vi "Auto1RecycleBin.vi"(8 "error in":errorcluster) -> ()   [LabVIEW 2014]
uses:
  <vilib>/Rock Robotics/WPI/DriverStation/WPI_DriverStationRobotMode2.ctl
  LowerLiftAndOpenArms.ctl
  Robot Global Data.vi
  Gantry/GantryGlobals.vi
  AutomationGlobals.vi
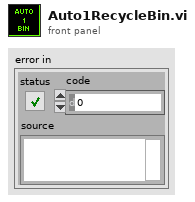
[diagram p1: front panel]
types:
  T1 = enum16{"WaitForInput", "GantryOut", "Lift", "Forward", "Autostack", "Left", "PutToteDown", "GrabBarrelLift", "Right", "Forward2", "Done"}
  T2 = typedef "WPI_DriverStationRobotMode2.ctl" = enum16{"Autonomous Disabled", "Autonomous Enabled", "Teleop Disabled", "Teleop Enabled", "Disconnected", "Finish", "Test Disabled", "Test Enabled", "Emergency Stopped"}
  T3 = typedef "LowerLiftAndOpenArms.ctl" = enum16{"WaitingForInput", "LowerLift", "OpenArms", "LowerLiftMore", "CloseArms", "RaiseLift", "StopArms"}
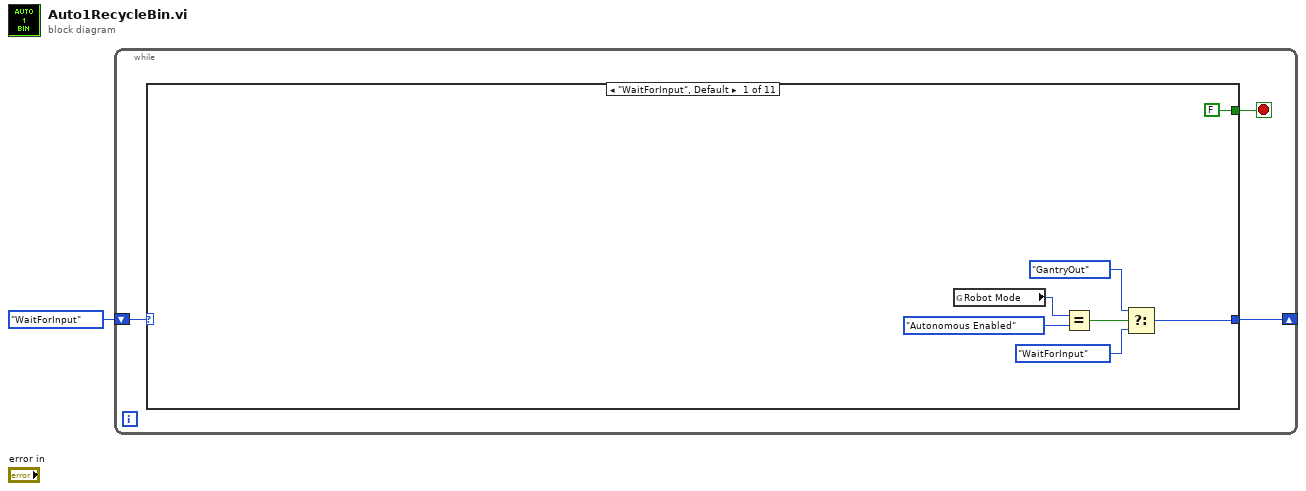
[diagram p0: block diagram]
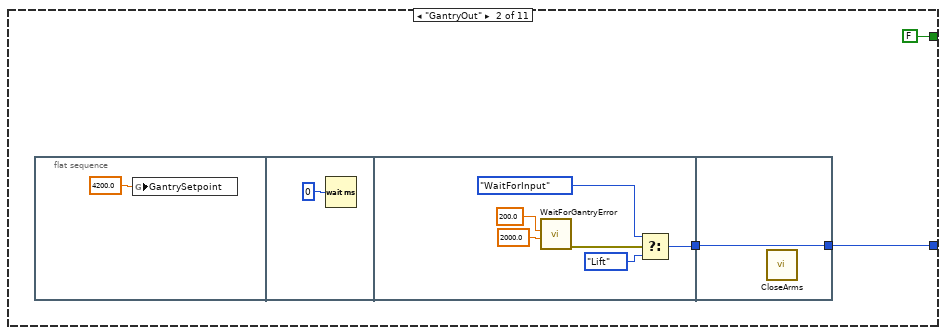
[diagram p2: hidden frame]
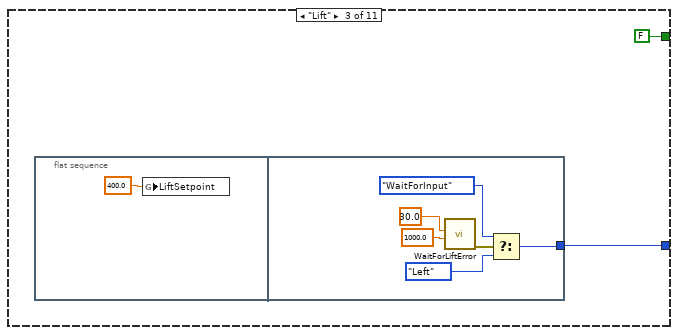
[diagram p3: hidden frame]
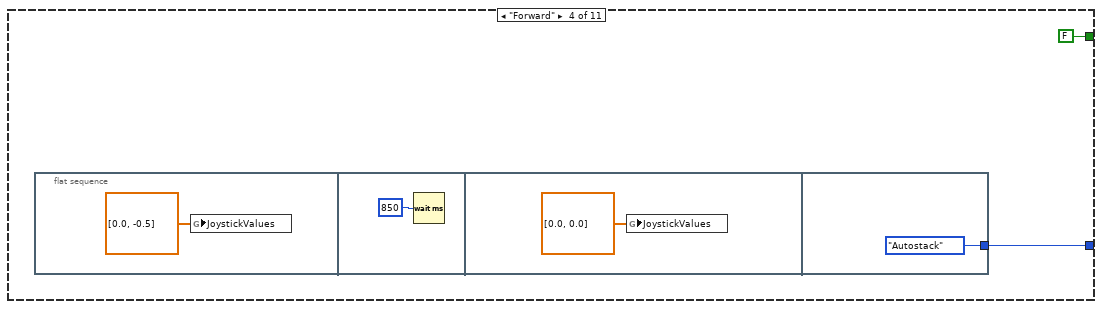
[diagram p4: hidden frame]
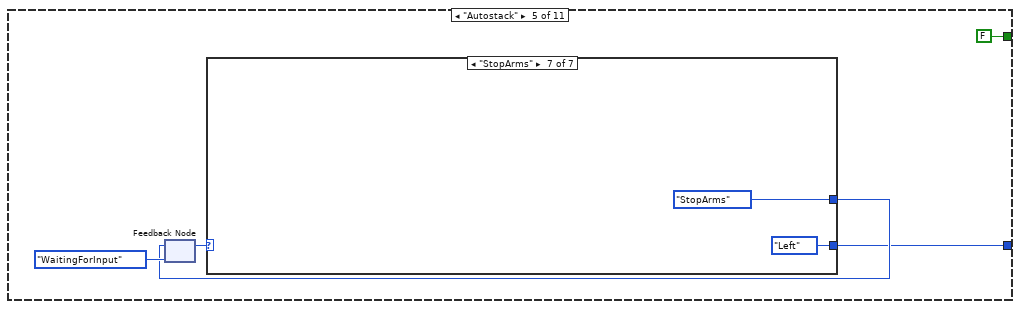
[diagram p5: hidden frame]
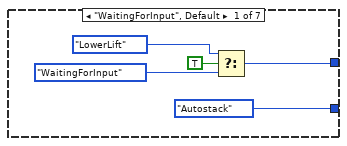
[diagram p6: hidden frame]
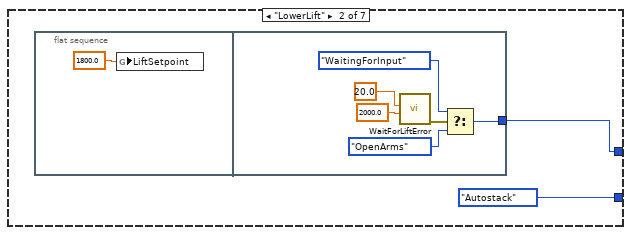
[diagram p7: hidden frame]
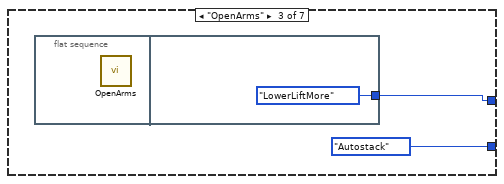
[diagram p8: hidden frame]
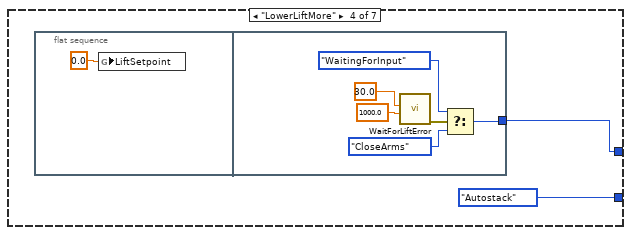
[diagram p9: hidden frame]
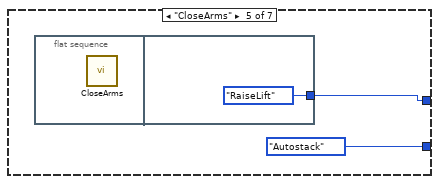
[diagram p10: hidden frame]
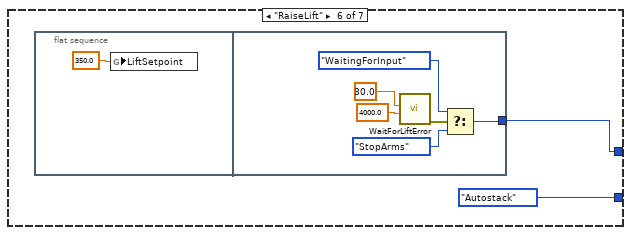
[diagram p11: hidden frame]
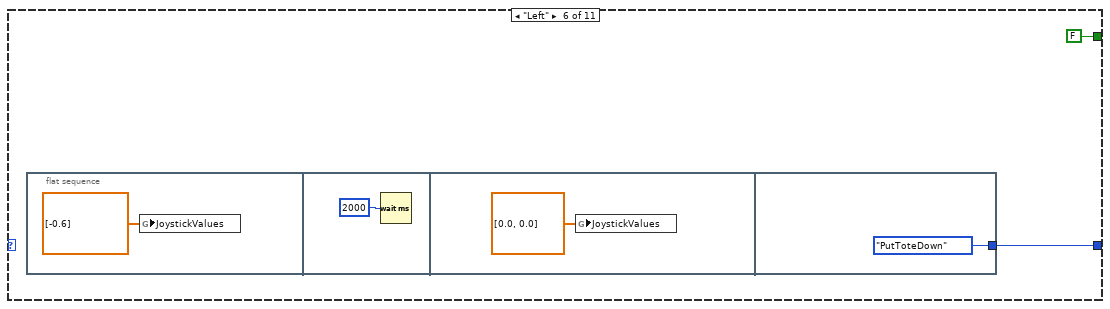
[diagram p12: hidden frame]
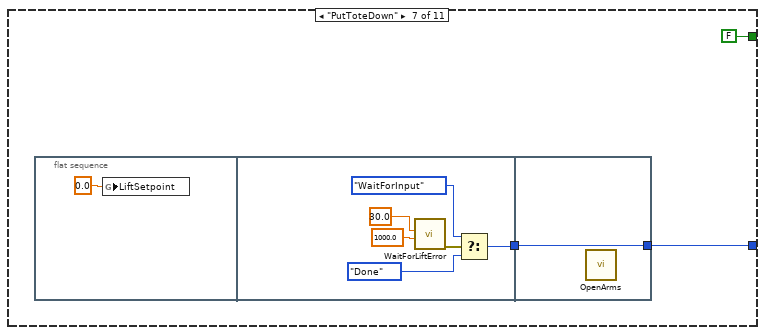
[diagram p13: hidden frame]
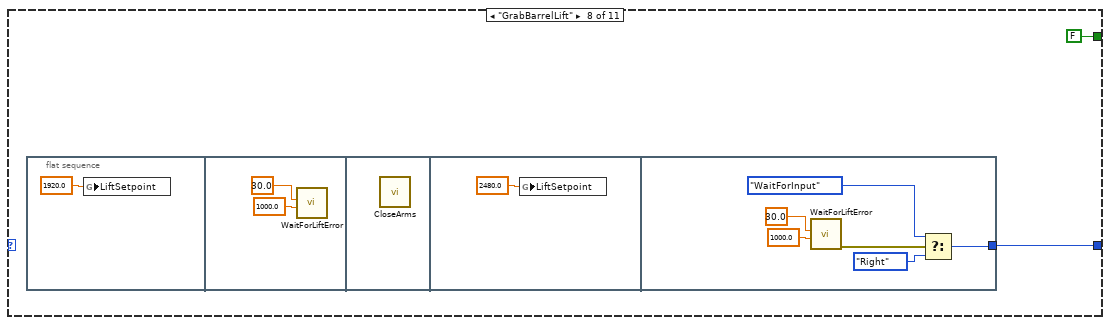
[diagram p14: hidden frame]
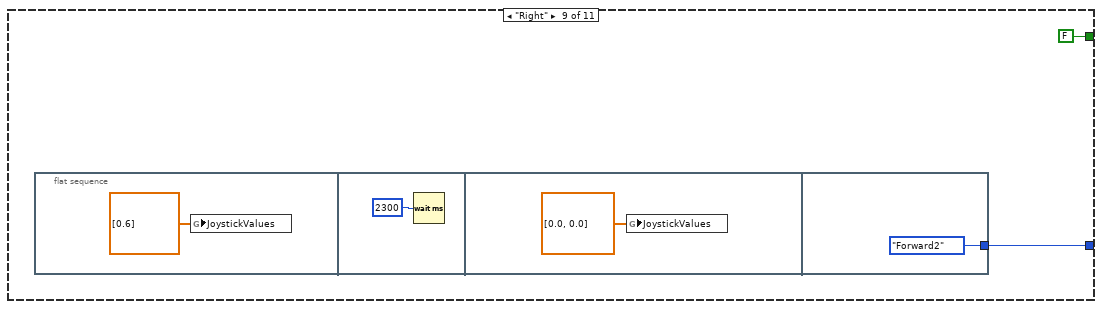
[diagram p15: hidden frame]
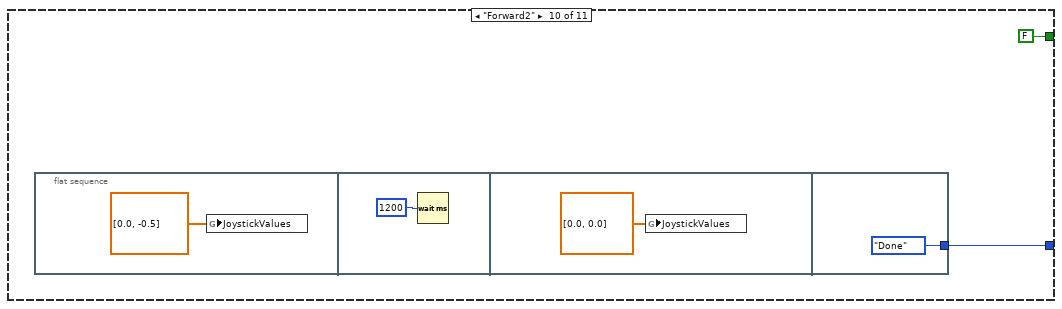
[diagram p16: hidden frame]
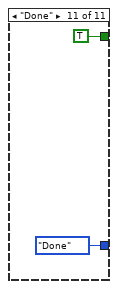
[diagram p17: hidden frame]
diagram:
  n1 = while {
    shift-right: [w3] -> _
    shift-left: T1."WaitForInput" ("Enum") -> [w4]
    stop <- w2 stop-if-true
    n2 = case shown="\"WaitForInput\", Default" w4 {
      tunnel: [w8 w14 w25 w33 w39 w84 w91 w101 w113 w120 T1."Done" ("Enum")] -> w3
      tunnel: [FALSE FALSE FALSE FALSE FALSE FALSE FALSE FALSE FALSE FALSE TRUE] -> w2
      frame "WaitForInput", Default {
        n3 = global read "Robot Global Data.vi" "Robot Mode"() -> (w11:T2)
        n4 = Equal?(x=w11, y=WPI_DriverStationRobotMode2."Autonomous Enabled") -> (x = y?=w9:bool)
        n5 = Select(t=T1."GantryOut" ("Enum"), s=w9, f=T1."WaitForInput" ("Enum")) -> (s? t:f=w8:T1)
      }
      frame "GantryOut" {
        n6 = flat-sequence {
          tunnel: [w19] -> w12
          tunnel: [w23] -> w14
          tunnel: w12 -> [w23]
          frame #0 {
            n7 = global write "GantryGlobals.vi" "GantrySetpoint"(4200.0 ("GantrySetpoint")) -> ()
          }
          frame #1 {
            n8 = Wait (ms)(milliseconds to wait=u32 0) -> ()  [unwired: 1 out]
          }
          frame #2 {
            n9 = call "WaitForGantryError.vi"("Timeout (ms)"=2000.0, "AllowedError"=200.0) -> ("error out"=w20:errorcluster)  [unwired: 9 in]
            n10 = Select(t=T1."WaitForInput" ("Enum"), s=w20, f=T1."Lift" ("Enum")) -> (s? t:f=w19:T1)
          }
          frame #3 {
            n11 = call "CloseArms.vi"() -> ()  [unwired: 12 in]
          }
        }
      }
      frame "Lift" {
        n12 = flat-sequence {
          tunnel: [w29] -> w25
          frame #0 {
            n13 = global write "GantryGlobals.vi" "LiftSetpoint"(400.0 ("LiftSetpoint")) -> ()
          }
          frame #1 {
            n14 = call "WaitForLiftError.vi"("Timeout (ms)"=1000.0, "AllowedError"=30.0) -> ("error out"=w32:errorcluster)  [unwired: 9 in]
            n15 = Select(t=T1."WaitForInput" ("Enum"), s=w32, f=T1."Left" ("Enum")) -> (s? t:f=w29:T1)
          }
        }
      }
      frame "Forward" {
        n16 = flat-sequence {
          tunnel: [T1."Autostack" ("Enum")] -> w33
          frame #0 {
            n17 = global write "AutomationGlobals.vi" "JoystickValues"(dbl[] [0.0, -0.5] ("s? t:f")) -> ()
          }
          frame #1 {
            n18 = Wait (ms)(milliseconds to wait=u32 850) -> ()  [unwired: 1 out]
          }
          frame #2 {
            n19 = global write "AutomationGlobals.vi" "JoystickValues"(dbl[] [0.0, 0.0] ("s? t:f")) -> ()
          }
          frame #3 {
          }
        }
      }
      frame "Autostack" {
        n20 = feedback #1(LowerLiftAndOpenArms."WaitingForInput" ("LowerAndOpen")) -> (w41:T3)
        n21 = case shown="\"StopArms\"" w41 {
          tunnel: [w46 w50 w59 w62 w71 w74 LowerLiftAndOpenArms."StopArms" ("LowerAndOpen")] -> w40
          tunnel: [T1."Autostack" ("Enum") T1."Autostack" ("Enum") T1."Autostack" ("Enum") T1."Autostack" ("Enum") T1."Autostack" ("Enum") T1."Autostack" ("Enum") T1."Left" ("Enum")] -> w39
          frame "WaitingForInput", Default {
            n22 = Select(t=LowerLiftAndOpenArms."LowerLift" ("LowerAndOpen"), s=TRUE, f=LowerLiftAndOpenArms."WaitingForInput" ("LowerAndOpen")) -> (s? t:f=w46:T3)
          }
          frame "LowerLift" {
            n23 = flat-sequence {
              tunnel: [w52] -> w50
              frame #0 {
                n24 = global write "GantryGlobals.vi" "LiftSetpoint"(1800.0 ("LiftSetpoint")) -> ()
              }
              frame #1 {
                n25 = call "WaitForLiftError.vi"("Timeout (ms)"=2000.0, "AllowedError"=20.0) -> ("error out"=w55:errorcluster)  [unwired: 9 in]
                n26 = Select(t=LowerLiftAndOpenArms."WaitingForInput" ("LowerAndOpen"), s=w55, f=LowerLiftAndOpenArms."OpenArms" ("LowerAndOpen")) -> (s? t:f=w52:T3)
              }
            }
          }
          frame "OpenArms" {
            n27 = flat-sequence {
              tunnel: [LowerLiftAndOpenArms."LowerLiftMore" ("LowerAndOpen")] -> w59
              frame #0 {
                n28 = call "OpenArms.vi"() -> ()  [unwired: 12 in]
              }
              frame #1 {
              }
            }
          }
          frame "LowerLiftMore" {
            n29 = flat-sequence {
              tunnel: [w64] -> w62
              frame #0 {
                n30 = global write "GantryGlobals.vi" "LiftSetpoint"(0.0 ("LiftSetpoint")) -> ()
              }
              frame #1 {
                n31 = call "WaitForLiftError.vi"("Timeout (ms)"=1000.0, "AllowedError"=30.0) -> ("error out"=w67:errorcluster)  [unwired: 9 in]
                n32 = Select(t=LowerLiftAndOpenArms."WaitingForInput" ("LowerAndOpen"), s=w67, f=LowerLiftAndOpenArms."CloseArms" ("LowerAndOpen")) -> (s? t:f=w64:T3)
              }
            }
          }
          frame "CloseArms" {
            n33 = flat-sequence {
              tunnel: [LowerLiftAndOpenArms."RaiseLift" ("LowerAndOpen")] -> w71
              frame #0 {
                n34 = call "CloseArms.vi"() -> ()  [unwired: 12 in]
              }
              frame #1 {
              }
            }
          }
          frame "RaiseLift" {
            n35 = flat-sequence {
              tunnel: [w76] -> w74
              frame #0 {
                n36 = global write "GantryGlobals.vi" "LiftSetpoint"(350.0 ("LiftSetpoint")) -> ()
              }
              frame #1 {
                n37 = call "WaitForLiftError.vi"("Timeout (ms)"=4000.0, "AllowedError"=30.0) -> ("error out"=w79:errorcluster)  [unwired: 9 in]
                n38 = Select(t=LowerLiftAndOpenArms."WaitingForInput" ("LowerAndOpen"), s=w79, f=LowerLiftAndOpenArms."StopArms" ("LowerAndOpen")) -> (s? t:f=w76:T3)
              }
            }
          }
          frame "StopArms" {
          }
        }
        n39 = feedback-in #1(w40) -> ()
      }
      frame "Left" {
        n40 = flat-sequence {
          tunnel: [T1."PutToteDown" ("Enum")] -> w84
          frame #0 {
            n41 = global write "AutomationGlobals.vi" "JoystickValues"(dbl[] [-0.6] ("s? t:f")) -> ()
          }
          frame #1 {
            n42 = Wait (ms)(milliseconds to wait=u32 2000) -> ()  [unwired: 1 out]
          }
          frame #2 {
            n43 = global write "AutomationGlobals.vi" "JoystickValues"(dbl[] [0.0, 0.0] ("s? t:f")) -> ()
          }
          frame #3 {
          }
        }
      }
      frame "PutToteDown" {
        n44 = flat-sequence {
          tunnel: [w96] -> w90
          tunnel: [w100] -> w91
          tunnel: w90 -> [w100]
          frame #0 {
            n45 = global write "GantryGlobals.vi" "LiftSetpoint"(0.0 ("LiftSetpoint")) -> ()
          }
          frame #1 {
            n46 = call "WaitForLiftError.vi"("Timeout (ms)"=1000.0, "AllowedError"=30.0) -> ("error out"=w99:errorcluster)  [unwired: 9 in]
            n47 = Select(t=T1."WaitForInput" ("Enum"), s=w99, f=T1."Done" ("Enum")) -> (s? t:f=w96:T1)
          }
          frame #2 {
            n48 = call "OpenArms.vi"() -> ()  [unwired: 12 in]
          }
        }
      }
      frame "GrabBarrelLift" {
        n49 = flat-sequence {
          tunnel: [w112] -> w101
          frame #0 {
            n50 = global write "GantryGlobals.vi" "LiftSetpoint"(1920.0 ("LiftSetpoint")) -> ()
          }
          frame #1 {
            n51 = call "WaitForLiftError.vi"("Timeout (ms)"=1000.0, "AllowedError"=30.0) -> ()  [unwired: 9 in, 1 out]
          }
          frame #2 {
            n52 = call "CloseArms.vi"() -> ()  [unwired: 12 in]
          }
          frame #3 {
            n53 = global write "GantryGlobals.vi" "LiftSetpoint"(2480.0 ("LiftSetpoint")) -> ()
          }
          frame #4 {
            n54 = call "WaitForLiftError.vi"("Timeout (ms)"=1000.0, "AllowedError"=30.0) -> ("error out"=w111:errorcluster)  [unwired: 9 in]
            n55 = Select(t=T1."WaitForInput" ("Enum"), s=w111, f=T1."Right" ("Enum")) -> (s? t:f=w112:T1)
          }
        }
      }
      frame "Right" {
        n56 = flat-sequence {
          tunnel: [T1."Forward2" ("Enum")] -> w113
          frame #0 {
            n57 = global write "AutomationGlobals.vi" "JoystickValues"(dbl[] [0.6] ("s? t:f")) -> ()
          }
          frame #1 {
            n58 = Wait (ms)(milliseconds to wait=u32 2300) -> ()  [unwired: 1 out]
          }
          frame #2 {
            n59 = global write "AutomationGlobals.vi" "JoystickValues"(dbl[] [0.0, 0.0] ("s? t:f")) -> ()
          }
          frame #3 {
          }
        }
      }
      frame "Forward2" {
        n60 = flat-sequence {
          tunnel: [T1."Done" ("Enum")] -> w120
          frame #0 {
            n61 = global write "AutomationGlobals.vi" "JoystickValues"(dbl[] [0.0, -0.5] ("s? t:f")) -> ()
          }
          frame #1 {
            n62 = Wait (ms)(milliseconds to wait=u32 1200) -> ()  [unwired: 1 out]
          }
          frame #2 {
            n63 = global write "AutomationGlobals.vi" "JoystickValues"(dbl[] [0.0, 0.0] ("s? t:f")) -> ()
          }
          frame #3 {
          }
        }
      }
      frame "Done" {
      }
    }
  }
